vi "Error Query.vi"(8 "error in (no error)":errorcluster, 11 "VISA resource name":refnum<visa-resource-name>) -> (0 "error out":errorcluster, 1 "Error Message":string, 2 "Error Number":i32, 3 "VISA resource name out":refnum<visa-resource-name>)   [LabVIEW 2013, in "TDK-Lambda Z.lvlib"]
doc: "Reads an error code and a message from the instrument's error queue (query SYST:ERR?\"). Any instrument error is passed to the \"error out\" cluster as a VISA custom error. \n\nNote: This VI is called automatically by most driver VIs so it is not usually necessary to call this in an application."
uses:
  TDK-Lambda Z.lvlib
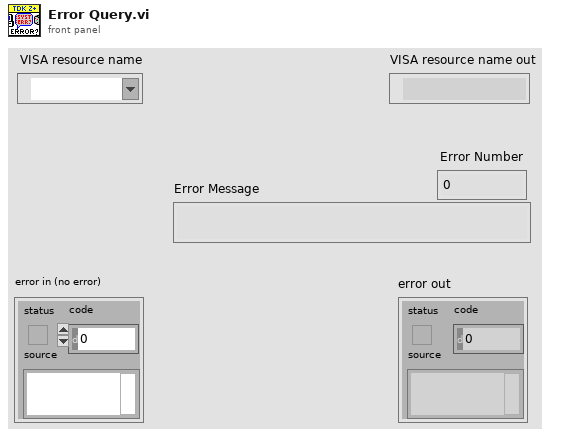
[diagram p1: front panel]
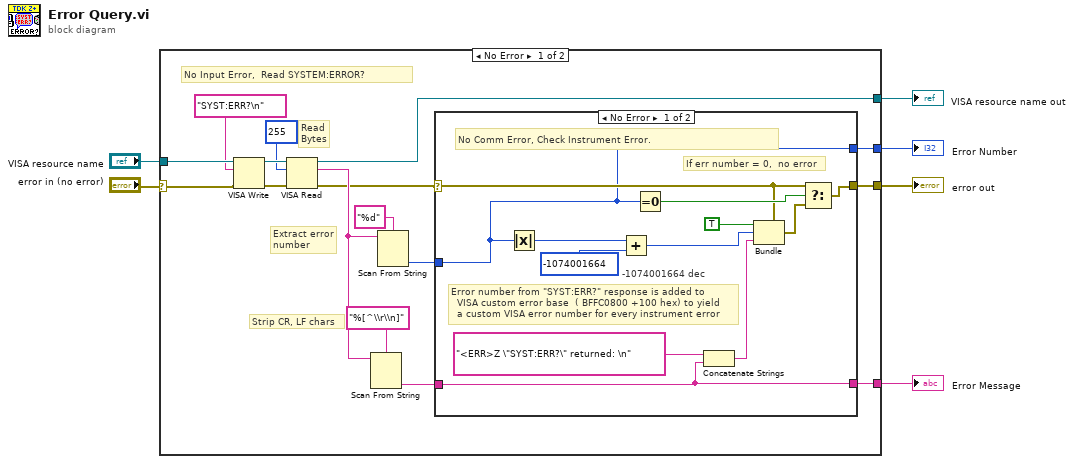
[diagram p0: block diagram]
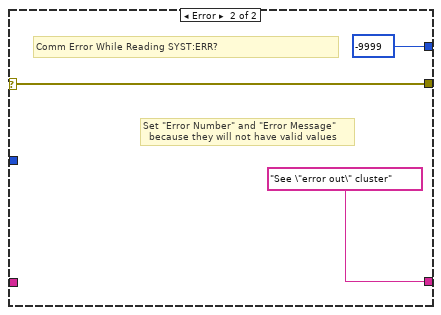
[diagram p2: hidden frame]
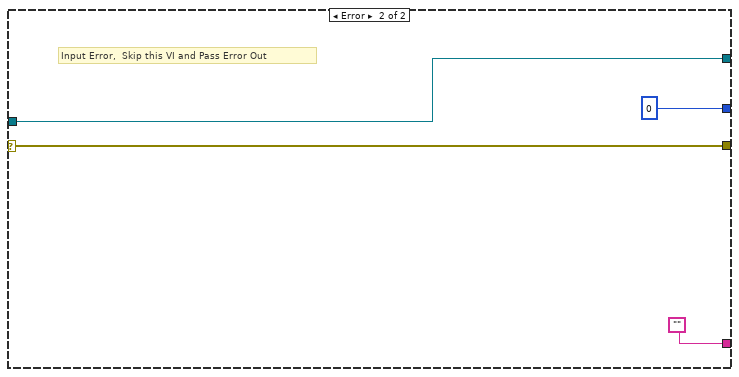
[diagram p3: hidden frame]
diagram:
  n1 = case shown="No Error" "error in (no error)" {
    selector: "error in (no error)" -> [w9 w38]
    tunnel: [w22 ""] -> w6
    tunnel: [w21 0] -> w5
    tunnel: [w7 w41] -> w4
    tunnel: "VISA resource name" -> [w20 w41]
    tunnel: [w10 w38] -> w2
    frame No Error {
      # "No Input Error,  Read SYSTEM:ERROR?"
      # "Extract error\nnumber"
      # "Read\nBytes"
      # "Strip CR, LF chars"
      n2 = VISA Write(VISA resource name=w20, write buffer="SYST:ERR?\n", error in (no error)=w9) -> (VISA resource name out=w19:refnum<visa-resource-name>, error out=w17:errorcluster)  [unwired: 1 out]
      n3 = VISA Read(VISA resource name=w19, byte count=u32 255 ("byte count (0)"), error in (no error)=w17) -> (VISA resource name out=w7:refnum<visa-resource-name>, read buffer=w12:string, error out=w8:errorcluster)  [unwired: 1 out]
      n4 = Scan From String(format string="%[^\\r\\n]", input string=w12) -> (output 1=w11:string)  [unwired: 3 in, 3 out]
      n5 = Scan From String(format string="%d", input string=w12) -> (output 1=w15:i32)  [unwired: 3 in, 3 out]
      n6 = case shown="No Error" w8 {
        selector: w8 -> [w27 w36]
        tunnel: [w31 w36] -> w10
        tunnel: [w28 "See \"error out\" cluster" ("format string")] -> w22
        tunnel: [w26 -9999] -> w21
        tunnel: w15 -> [w26 _]
        tunnel: w11 -> [w28 _]
        frame No Error {
          # "No Comm Error, Check Instrument Error."
          # "Error number from \"SYST:ERR?\" response is added to \n  VISA custom error base  ( BFFC0800 +100 hex) to yield  \n  a custom VISA error number for every instrument error"
          # "-1074001664 dec"
          # "If err number = 0,  no error"
          n7 = Absolute Value(x=w26) -> (abs(x)=w25:i32)
          n8 = Add(x=w25, y=-1074001664) -> (x+y=w23:i32)
          n9 = Equal To 0?(x=w26) -> (x = 0?=w29:bool)
          n10 = Concatenate Strings("<ERR>Z \"SYST:ERR?\" returned: \n" ("Source"), w28) -> (w33:string)
          n11 = Bundle(cluster=w27, "status"=TRUE ("Status"), "code"=w23, "source"=w33) -> (w32:errorcluster)
          n12 = Select(t=w27, s=w29, f=w32) -> (s? t:f=w31:errorcluster)
        }
        frame Error {
          # "Set \"Error Number\" and \"Error Message\"\n  because they will not have valid values"
          # "Comm Error While Reading SYST:ERR?"
        }
      }
    }
    frame Error {
      # "Input Error,  Skip this VI and Pass Error Out"
    }
  }
  "Error Message" <- w6
  "Error Number" <- w5
  "VISA resource name out" <- w4
  "error out" <- w2
